vi "Finish.vi"   [LabVIEW 2018]
doc: "This VI is called just before exiting. It is expected to close I/O refnum, save collected data, etc."
uses:
  <vilib>/Rock Robotics/WPI/Utilities/WPI_GetSetVariantRefNum.vi
types:
  T1 = typedef "WPI_MotorControlDeviceRef.ctl" = cluster{"DeviceStatus":errorcluster, "Type":T2, "PWM":cluster{"PWM Channel":T3, "DeadBand":T4}, "CAN":cluster{"Device Number":u8, "SetOutput VI Ref":variant, "GetOutput VI Ref":variant, "Enable VI Ref":variant, "Disable VI Ref":variant, "Data":variant}, "Invert":bool, "DIO PWM":cluster{"PWM \"Enable\" Channel":T3, "DIOChannel":T5, "PWM Rate":dbl}}
  T2 = typedef "WPI_MotorControlType.ctl" = enum16{"PWM", "CAN", "DIO PWM"}
  T3 = typedef "FPGA_DIOPWMChannel.ctl" = enum8{"PWM 0", "PWM 1", "PWM 2", "PWM 3", "PWM 4", "PWM 5", "PWM 6", "PWM 7", "PWM 8", "PWM 9", "PWM MXP 0", "PWM MXP 1", "PWM MXP 2", "PWM MXP 3", "PWM MXP 4", "PWM MXP 5", "PWM MXP 6", "PWM MXP 7", "PWM MXP 8", "PWM MXP 9", "Invalid"}
  T4 = typedef "WPI_PWMDeadband.ctl" = cluster{"Name":string, "maxPositivePwm":i32, "minPositivePwm":i32, "centerPwm":i32, "maxNegativePwm":i32, "minNegativePwm":i32, "angularRange":u16}
  T5 = typedef "FPGA_DIOChannel.ctl" = enum8{"DIO 0", "DIO 1", "DIO 2", "DIO 3", "DIO 4", "DIO 5", "DIO 6", "DIO 7", "DIO 8", "DIO 9", "DIO MXP 0", "DIO MXP 1", "DIO MXP 2", "DIO MXP 3", "DIO MXP 4", "DIO MXP 5", "DIO MXP 6", "DIO MXP 7", "DIO MXP 8", "DIO MXP 9", "DIO MXP 10", "DIO MXP 11", "DIO MXP 12", "DIO MXP 13", "DIO MXP 14", "DIO MXP 15", "SPI Port CS1", "SPI Port CS2", "SPI Port CS3", "SPI Port MISO", "SPI Port MOSI", "Invalid"}
  T6 = typedef "WPI_SolenoidDevRef.ctl" = cluster{"DevStatus":errorcluster, "Pneumatics Control Module":u8, "Forward Solenoid Channel":T7, "Reverse Solenoid Channel":T7}
  T7 = typedef "WPI_SolenoidChannel.ctl" = enum8{"Solenoid 0", "Solenoid 1", "Solenoid 2", "Solenoid 3", "Solenoid 4", "Solenoid 5", "Solenoid 6", "Solenoid 7", "Invalid"}
  T8 = typedef "WPI_JoystickDevRef.ctl" = cluster{"Device":T9}
  T9 = typedef "WPI_JoystickDeviceEnum.ctl" = enum16{"USB 0", "USB 1", "USB 2", "USB 3", "USB 4", "USB 5"}
  T10 = typedef "WPI_EncoderDevRef.ctl" = cluster{"DevStatus":errorcluster, "EncoderIndex":T11, "CounterIndex":T12, "DistancePerCount":dbl, "Decoding Type":T13}
  T11 = typedef "FPGA_EncoderIdx.ctl" = enum8{"Enc 0", "Enc 1", "Enc 2", "Enc 3", "Enc 4", "Enc 5", "Enc 6", "Enc 7", "Invalid"}
  T12 = typedef "FPGA_CounterCtrSystemIndex.ctl" = enum8{"Ctr 0", "Ctr 1", "Ctr 2", "Ctr 3", "Ctr 4", "Ctr 5", "Ctr 6", "Ctr 7", "Invalid"}
  T13 = typedef "WPI_EncoderType.ctl" = enum16{"1x", "2x", "4x"}
  T14 = typedef "WPI_CompressorDevRef.ctl" = cluster{"DevStatus":errorcluster, "Pneumatics Control Module":u8}
  T15 = typedef "WPI_PotentiometerDevRef.ctl" = cluster{"DevStatus":errorcluster, "Analog Channel":T16, "Invert Output":bool}
  T16 = typedef "FPGA_AIChannel.ctl" = enum8{"AI 0", "AI 1", "AI 2", "AI 3", "AI MXP 0", "AI MXP 1", "AI MXP 2", "AI MXP 3", "Invalid"}
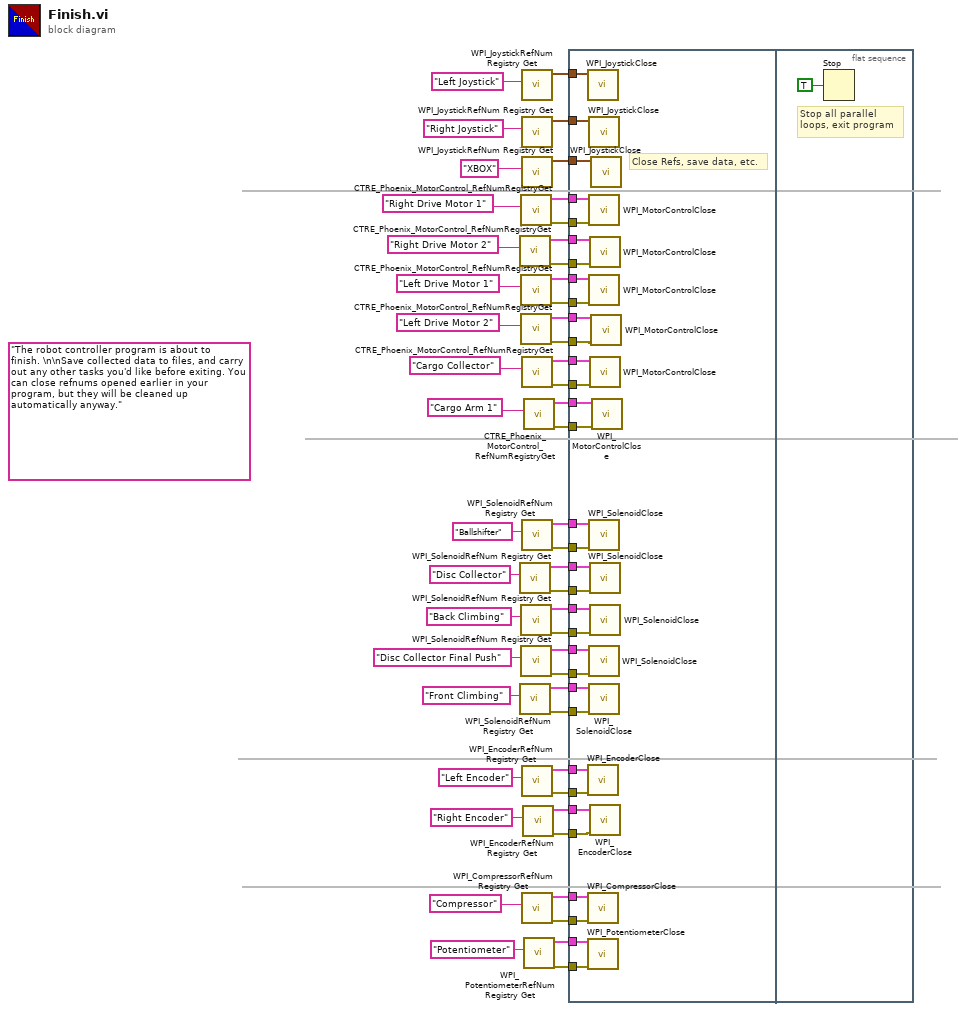
[diagram p0: block diagram]
diagram:
  (unwired) "The robot controller program is about to finish. \n\nSave collected data to files, and carry out any other tasks you'd like before exiting. You can close refnums opened earlier in your program, but they will be cleaned up automatically anyway."
  n1 = call <vilib>:"CTRE_Phoenix_MotorControl_RefNumRegistryGet.vi"("refnum name"="Right Drive Motor 2") -> ("error out"=w37:errorcluster, "PhoenixMotorControlDevRef"=w38:T1)  [unwired: 9 in]
  n2 = call <vilib>:"WPI_SolenoidRefNum Registry Get.vi"("refnum name"="Disc Collector") -> ("error out"=w21:errorcluster, "SolenoidDevRef"=w22:T6)  [unwired: 9 in]
  n3 = call <vilib>:"WPI_SolenoidRefNum Registry Get.vi"("refnum name"="Front Climbing") -> ("error out"=w15:errorcluster, "SolenoidDevRef"=w16:T6)  [unwired: 9 in]
  n4 = call <vilib>:"CTRE_Phoenix_MotorControl_RefNumRegistryGet.vi"("refnum name"="Right Drive Motor 1") -> ("error out"=w41:errorcluster, "PhoenixMotorControlDevRef"=w42:T1)  [unwired: 9 in]
  n5 = call <vilib>:"CTRE_Phoenix_MotorControl_RefNumRegistryGet.vi"("refnum name"="Left Drive Motor 1") -> ("error out"=w31:errorcluster, "PhoenixMotorControlDevRef"=w32:T1)  [unwired: 9 in]
  n6 = call <vilib>:"CTRE_Phoenix_MotorControl_RefNumRegistryGet.vi"("refnum name"="Left Drive Motor 2") -> ("error out"=w29:errorcluster, "PhoenixMotorControlDevRef"=w30:T1)  [unwired: 9 in]
  n7 = call <vilib>:"WPI_SolenoidRefNum Registry Get.vi"("refnum name"="Back Climbing") -> ("error out"=w19:errorcluster, "SolenoidDevRef"=w20:T6)  [unwired: 9 in]
  n8 = call <vilib>:"WPI_SolenoidRefNum Registry Get.vi"("refnum name"="Disc Collector Final Push") -> ("error out"=w17:errorcluster, "SolenoidDevRef"=w18:T6)  [unwired: 9 in]
  n9 = call <vilib>:"WPI_JoystickRefNum Registry Get.vi"("refnum name"="Left Joystick") -> ("JoystickDevRef"=w47:T8)  [unwired: 1 in, 9 out]
  n10 = call <vilib>:"WPI_JoystickRefNum Registry Get.vi"("refnum name"="Right Joystick") -> ("JoystickDevRef"=w46:T8)  [unwired: 1 in, 9 out]
  n11 = call <vilib>:"WPI_JoystickRefNum Registry Get.vi"("refnum name"="XBOX") -> ("JoystickDevRef"=w50:T8)  [unwired: 1 in, 9 out]
  n12 = call <vilib>:"CTRE_Phoenix_MotorControl_RefNumRegistryGet.vi"("refnum name"="Cargo Collector") -> ("error out"=w27:errorcluster, "PhoenixMotorControlDevRef"=w28:T1)  [unwired: 9 in]
  n13 = call <vilib>:"WPI_SolenoidRefNum Registry Get.vi"("refnum name"="Ballshifter") -> ("error out"=w23:errorcluster, "SolenoidDevRef"=w24:T6)  [unwired: 9 in]
  n14 = call <vilib>:"WPI_EncoderRefNum Registry Get.vi"("refnum name"="Left Encoder") -> ("error out"=w8:errorcluster, "EncoderDevRef"=w9:T10)  [unwired: 9 in]
  n15 = call <vilib>:"WPI_CompressorRefNum Registry Get.vi"("refnum name"="Compressor") -> ("error out"=w45:errorcluster, "CompressorDevRef"=w44:T14)  [unwired: 9 in]
  n16 = call <vilib>:"WPI_EncoderRefNum Registry Get.vi"("refnum name"="Right Encoder") -> ("error out"=w4:errorcluster, "EncoderDevRef"=w5:T10)  [unwired: 9 in]
  n17 = call <vilib>:"CTRE_Phoenix_MotorControl_RefNumRegistryGet.vi"("refnum name"="Cargo Arm 1") -> ("error out"=w25:errorcluster, "PhoenixMotorControlDevRef"=w26:T1)  [unwired: 9 in]
  n18 = call <vilib>:"WPI_PotentiometerRefNum Registry Get.vi"("refnum name"="Potentiometer") -> ("error out"=w2:errorcluster, "PotDevRef"=w3:T15)  [unwired: 9 in]
  n19 = flat-sequence {
    tunnel: w50 -> [w84]
    tunnel: w47 -> [w83]
    tunnel: w46 -> [w82]
    tunnel: w45 -> [w81]
    tunnel: w44 -> [w80]
    tunnel: w42 -> [w79]
    tunnel: w41 -> [w78]
    tunnel: w38 -> [w77]
    tunnel: w37 -> [w76]
    tunnel: w32 -> [w75]
    tunnel: w31 -> [w74]
    tunnel: w30 -> [w73]
    tunnel: w29 -> [w72]
    tunnel: w28 -> [w71]
    tunnel: w27 -> [w70]
    tunnel: w26 -> [w69]
    tunnel: w25 -> [w68]
    tunnel: w24 -> [w67]
    tunnel: w23 -> [w66]
    tunnel: w22 -> [w65]
    tunnel: w21 -> [w64]
    tunnel: w20 -> [w63]
    tunnel: w19 -> [w62]
    tunnel: w18 -> [w61]
    tunnel: w17 -> [w60]
    tunnel: w16 -> [w59]
    tunnel: w15 -> [w58]
    tunnel: w9 -> [w57]
    tunnel: w8 -> [w56]
    tunnel: w5 -> [w55]
    tunnel: w4 -> [w54]
    tunnel: w3 -> [w53]
    tunnel: w2 -> [w52]
    frame #0 {
      # "Close Refs, save data, etc."
      n20 = call <vilib>:"WPI_JoystickClose.vi"("JoystickDevRef"=w83) -> ()  [unwired: 11 out]
      n21 = call <vilib>:"WPI_EncoderClose.vi"("error in (no error)"=w56, "EncoderDevRef"=w57) -> ()  [unwired: 9 in, 1 out]
      n22 = call <vilib>:"WPI_CompressorClose.vi"("error in (no error)"=w81, "CompressorDevRef"=w80) -> ()  [unwired: 9 in, 1 out]
      n23 = call <vilib>:"WPI_PotentiometerClose.vi"("error in"=w52, "PotDevRef"=w53) -> ()  [unwired: 9 in, 1 out]
      n24 = call <vilib>:"WPI_JoystickClose.vi"("JoystickDevRef"=w82) -> ()  [unwired: 11 out]
      n25 = call <vilib>:"WPI_MotorControlClose.vi"("error in"=w78, "MotorControlDevRef"=w79) -> ()  [unwired: 9 in, 1 out]
      n26 = call <vilib>:"WPI_MotorControlClose.vi"("error in"=w74, "MotorControlDevRef"=w75) -> ()  [unwired: 9 in, 1 out]
      n27 = call <vilib>:"WPI_SolenoidClose.vi"("error in (no error)"=w66, "SolenoidDevRef"=w67) -> ()  [unwired: 9 in, 1 out]
      n28 = call <vilib>:"WPI_SolenoidClose.vi"("error in (no error)"=w60, "SolenoidDevRef"=w61) -> ()  [unwired: 9 in, 1 out]
      n29 = call <vilib>:"WPI_SolenoidClose.vi"("error in (no error)"=w58, "SolenoidDevRef"=w59) -> ()  [unwired: 9 in, 1 out]
      n30 = call <vilib>:"WPI_MotorControlClose.vi"("error in"=w76, "MotorControlDevRef"=w77) -> ()  [unwired: 9 in, 1 out]
      n31 = call <vilib>:"WPI_MotorControlClose.vi"("error in"=w70, "MotorControlDevRef"=w71) -> ()  [unwired: 9 in, 1 out]
      n32 = call <vilib>:"WPI_SolenoidClose.vi"("error in (no error)"=w64, "SolenoidDevRef"=w65) -> ()  [unwired: 9 in, 1 out]
      n33 = call <vilib>:"WPI_SolenoidClose.vi"("error in (no error)"=w62, "SolenoidDevRef"=w63) -> ()  [unwired: 9 in, 1 out]
      n34 = call <vilib>:"WPI_EncoderClose.vi"("error in (no error)"=w54, "EncoderDevRef"=w55) -> ()  [unwired: 9 in, 1 out]
      n35 = call <vilib>:"WPI_JoystickClose.vi"("JoystickDevRef"=w84) -> ()  [unwired: 11 out]
      n36 = call <vilib>:"WPI_MotorControlClose.vi"("error in"=w72, "MotorControlDevRef"=w73) -> ()  [unwired: 9 in, 1 out]
      n37 = call <vilib>:"WPI_MotorControlClose.vi"("error in"=w68, "MotorControlDevRef"=w69) -> ()  [unwired: 9 in, 1 out]
    }
    frame #1 {
      # "Stop all parallel\nloops, exit program"
      n38 = Stop(stop? (T)=TRUE ("Quit")) -> ()
    }
  }
